vi "VI Tree.vi"   [LabVIEW 2015, in "RIGOL DS1000 Series.lvlib"]
doc: "This is the instrument driver for the DS1000B DS1000E DS1000CA DS1000U DS1000D Series Digital Oscilloscopes. The VI Tree displays all the user-callable VIs of the instrument driver in an organized table."
uses:
  RIGOL DS1000 Series.lvlib
  Data/Read (Single Waveform).vi
  Configure/Configure Trigger (Edge).vi
panel:
  # "(c) 2010-2012, RIGOL Technologies, Inc.  All Rights Reserved."
  # "SEE DIAGRAM\nFOR VI TREE."
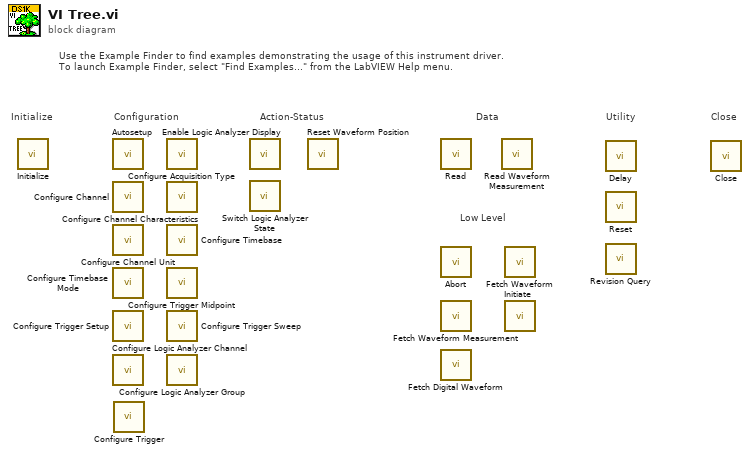
[diagram p0: block diagram]
diagram:
  # "Action-Status"
  # "Low Level"
  # "Use the Example Finder to find examples demonstrating the usage of this instrument driver.\nTo launch Example Finder, select \"Find Examples...\" from the LabVIEW Help menu."
  # "Configuration"
  # "Utility"
  # "Data"
  # "Close"
  # "Initialize"
  n1 = call "Initialize.vi"() -> ()  [unwired: 10 in, 2 out]
  n2 = call "Autosetup.vi"() -> ()  [unwired: 10 in, 2 out]
  n3 = call "Configure Channel.vi"() -> ()  [unwired: 14 in, 2 out]
  n4 = call "Configure Channel Unit.vi"() -> ()  [unwired: 10 in, 2 out]
  n5 = call "Configure Timebase Mode.vi"() -> ()  [unwired: 10 in, 2 out]
  n6 = call "Configure Trigger Setup.vi"() -> ()  [unwired: 10 in, 2 out]
  n7 = call "Configure Logic Analyzer Channel.vi"() -> ()  [unwired: 10 in, 2 out]
  n8 = call-poly "Configure Trigger.vi"() -> ()  [unwired: 14 in, 2 out]
  n9 = call "Configure Acquisition Type.vi"() -> ()  [unwired: 10 in, 2 out]
  n10 = call "Configure Channel Characteristics.vi"() -> ()  [unwired: 10 in, 2 out]
  n11 = call "Configure Timebase.vi"() -> ()  [unwired: 10 in, 2 out]
  n12 = call "Configure Trigger Midpoint.vi"() -> ()  [unwired: 10 in, 2 out]
  n13 = call "Configure Trigger Sweep.vi"() -> ()  [unwired: 10 in, 2 out]
  n14 = call "Configure Logic Analyzer Group.vi"() -> ()  [unwired: 10 in, 2 out]
  n15 = call "Enable Logic Analyzer Display.vi"() -> ()  [unwired: 10 in, 2 out]
  n16 = call "Switch Logic Analyzer State.vi"() -> ()  [unwired: 10 in, 2 out]
  n17 = call "Reset Waveform Position.vi"() -> ()  [unwired: 10 in, 2 out]
  n18 = call-poly "Read.vi"() -> ()  [unwired: 9 in, 3 out]
  n19 = call "Abort.vi"() -> ()  [unwired: 10 in, 2 out]
  n20 = call "Fetch Waveform Measurement.vi"() -> ()  [unwired: 9 in, 3 out]
  n21 = call "Fetch Digital Waveform.vi"() -> ()  [unwired: 9 in, 3 out]
  n22 = call "Read Waveform Measurement.vi"() -> ()  [unwired: 9 in, 3 out]
  n23 = call "Fetch Waveform.vi"() -> ()  [unwired: 9 in, 3 out]
  n24 = call "Initiate.vi"() -> ()  [unwired: 10 in, 2 out]
  n25 = call "Delay.vi"() -> ()  [unwired: 10 in, 2 out]
  n26 = call "Reset.vi"() -> ()  [unwired: 10 in, 2 out]
  n27 = call "Revision Query.vi"() -> ()  [unwired: 8 in, 4 out]
  n28 = call "Close.vi"() -> ()  [unwired: 11 in, 1 out]
